vi "Init DUT.vi"(8 "error in (no error)":errorcluster, 10 "DUT HW Resources":T1={"CAN Interface"="CAN2", "CAN Termination"=TRUE, "Digital Counter"="Dev1/ctr0", "DO Terminals"=[]}, 11 "DUT Sample in":refnum<class "DUT Sample.lvclass">) -> (0 "error out":errorcluster, 3 "DUT Sample out":refnum<class "DUT Sample.lvclass">)   [LabVIEW 2023, in "DUT Sample.lvclass"]
uses:
  DUT Sample.lvclass
  DUT Sample.lvclass/DUT Sample.ctl
  typedefs/DUT HW Resources.ctl
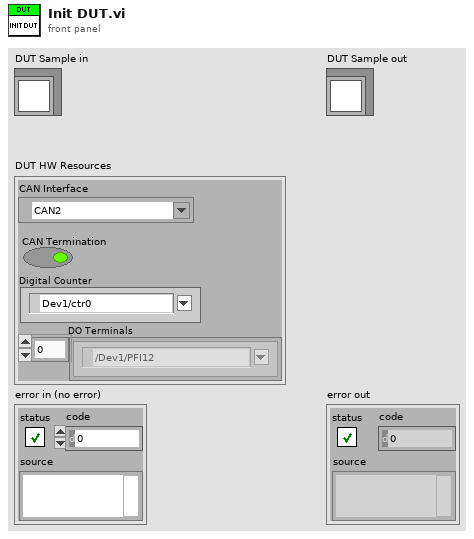
[diagram p1: front panel]
types:
  T1 = typedef "DUT Sample.lvclass/DUT HW Resources.ctl" = cluster{"CAN Interface":refnum<k21>, "CAN Termination":bool, "Digital Counter":tag, "DO Terminals":tag[]}
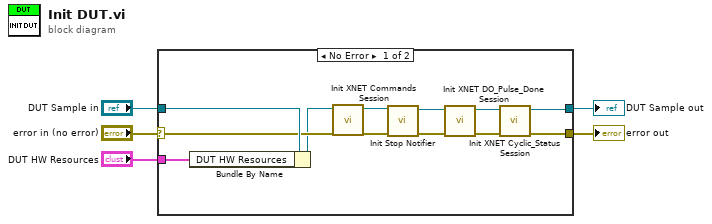
[diagram p0: block diagram]
diagram:
  n1 = case shown="No Error" "error in (no error)" {
    selector: "error in (no error)" -> [w16 w19]
    tunnel: [w8 w19] -> w4
    tunnel: [w6 w18] -> w2
    tunnel: "DUT Sample in" -> [w17 w18]
    tunnel: "DUT HW Resources" -> [w11 _]
    frame No Error {
      n2 = Bundle By Name(cluster=w17, "DUT HW Resources"=w11) -> (w12:refnum<class "DUT Sample.lvclass">)
      n3 = call "Init XNET Commands Session.vi"("error in (no error)"=w16, "DUT Sample in"=w12) -> ("error out"=w15:errorcluster, "DUT Sample out"=w13:refnum<class "DUT Sample.lvclass">)  [unwired: 8 in]
      n4 = call "Init Stop Notifier.vi"("error in (no error)"=w15, "DUT Sample in"=w13) -> ("error out"=w14:errorcluster, "DUT Sample out"=w9:refnum<class "DUT Sample.lvclass">)  [unwired: 8 in]
      n5 = call "Init XNET DO_Pulse_Done Session.vi"("error in (no error)"=w14, "DUT Sample in"=w9) -> ("error out"=w10:errorcluster, "DUT Sample out"=w7:refnum<class "DUT Sample.lvclass">)  [unwired: 8 in]
      n6 = call "Init XNET Cyclic_Status Session.vi"("error in (no error)"=w10, "DUT Sample in"=w7) -> ("error out"=w8:errorcluster, "DUT Sample out"=w6:refnum<class "DUT Sample.lvclass">)  [unwired: 8 in]
    }
    frame Error {
    }
  }
  "error out" <- w4
  "DUT Sample out" <- w2
